vi "ModemTest4.vi"() -> ()   [LabVIEW 2010]
panel:
  out "# elements in queue":i32
  out "Length":i32
  out "Output":string
  in  "stop":bool
  out "Encoded Data Out":u8[](array[numeric])
  out "Voltage":u8
  out "Current":u8
  out "Capacity":i16
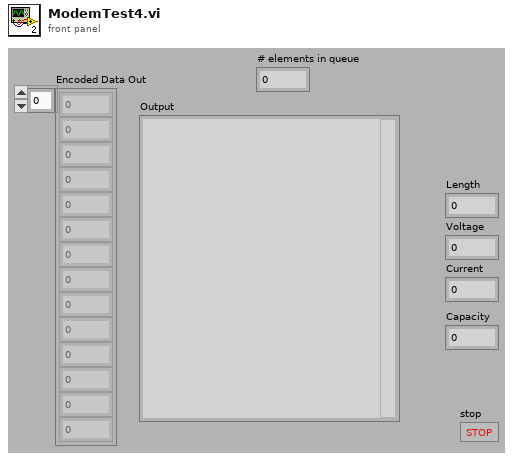
[diagram p1: front panel]
types:
  T1 = typedef "ModemTelemetryPacket.ctl" = cluster{"id":i16, "latitude":i32, "longitude":i32, "altitude":i16, "course":i16, "heading":i16, "speed":i16, "voltage":u8, "current":u8, "capacity":i16, "reserved":i16, "ecc":u8[]}
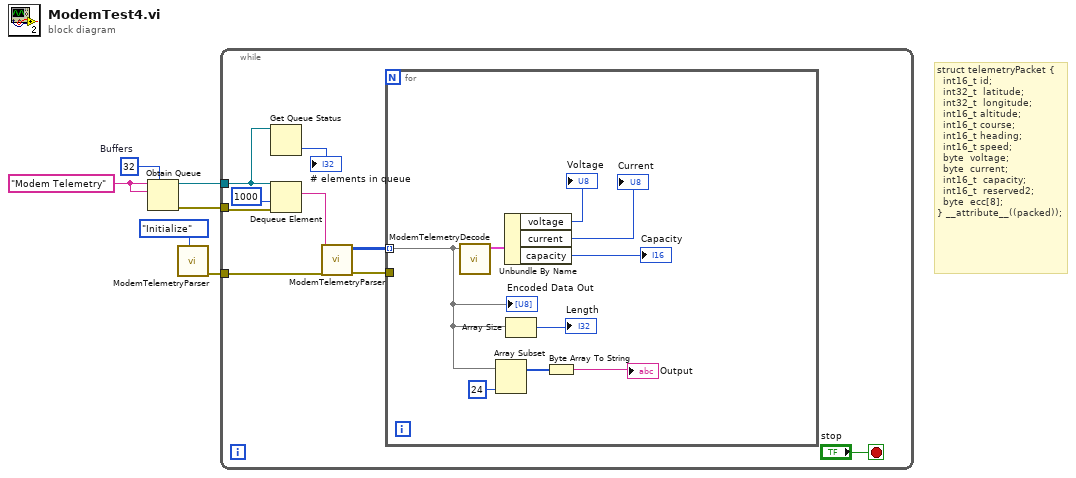
[diagram p0: block diagram]
diagram:
  w6 = 32  # Buffers
  w3 = "Modem Telemetry" ("name (unnamed)")
  # "struct telemetryPacket {\n  int16_t id;\n  int32_t  latitude;\n  int32_t  longitude;\n  int16_t altitude;\n  int16_t course;\n  int16_t heading;\n  int16_t speed;\n  byte  voltage;\n  byte  current;\n  int16_t  capacity;\n  int16_t  reserved2;\n  byte  ecc[8];\n} __attribute__((packed));"
  n1 = Obtain Queue(max queue size (-1, unlimited)=w6, name (unnamed)=w3, element data type=w3) -> (queue out=w5:refnum<queue>, error out=w4:errorcluster)  [unwired: 2 in, 1 out]
  n2 = call "ModemTelemetryParser.vi"("Operation"=enum16{"Parse", "Initialize"}."Initialize") -> ("Error Out"=w1:errorcluster)  [unwired: 9 in, 1 out]
  n3 = while {
    tunnel: w5 -> [w8]
    tunnel: w4 -> [w14]
    tunnel: w1 -> [w13]
    stop <- "stop" stop-if-true
    n4 = Get Queue Status(queue=w8) -> (# elements in queue=→"# elements in queue":i32)  [unwired: 2 in, 7 out]
    n5 = Dequeue Element(queue=w8, timeout in ms (-1)=1000, error in (no error)=w14) -> (element=w12:string)  [unwired: 3 out]
    n6 = call "ModemTelemetryParser.vi"("Error In"=w13, "Serial Data In"=w12) -> ("Error Out"=w10:errorcluster, "Detected Frames"=w11:u8[][])  [unwired: 8 in]
    n7 = for {
      tunnel: w11 -> [w24] mode=indexing
      tunnel: w10 -> [_]
      n8 = call "ModemTelemetryDecode.vi"("Encoded Data"=w24) -> ("TelemetryPacket"=w23:T1)  [unwired: 9 in, 1 out]
      n9 = Array Subset(array=w24, length=24) -> (w18:u8[])  [unwired: 1 in]
      n10 = Unbundle By Name(w23) -> ("voltage"=→"Voltage":u8, "current"=→"Current":u8, "capacity"=→"Capacity":i16)
      n11 = Array Size(array=w24) -> (size(s)=→"Length":i32)
      n12 = Byte Array To String(unsigned byte array=w18) -> (string=→"Output":string)
      "Encoded Data Out" <- w24
    }
  }
